vi "zmq_data_server.vi"() -> ()   [LabVIEW 2013]
doc: "Sends a specified waveform through a TCP port. The VI first listens for a connection and, once established, sends the number of bytes to be sent followed by the data. After the data is sent, the VI waits for an 'all received' signal from the client and then breaks the connection.\n\n<B>Note:</B> Requires the Data Client.vi located in the same library as this VI."
uses:
  <vilib>/addons/zeromq/socket_type.ctl
panel:
  in  "amplitude period (ms)":u32
  out "Waveform Graph":dbl[](graph)
  out "*(type *) &x":string
  in  "stop":bool
  in  "Noise Level":dbl(slide)=0.36734693877551017 scale=0.0..1.0 scale format="%0.1f"
  in  "# of Points":i32=200
  in  "Function":u16(ring)=1 items=["random", "sine wave", "cosine wave"]
  in  "Port":u16=6340 min=1025 step=1
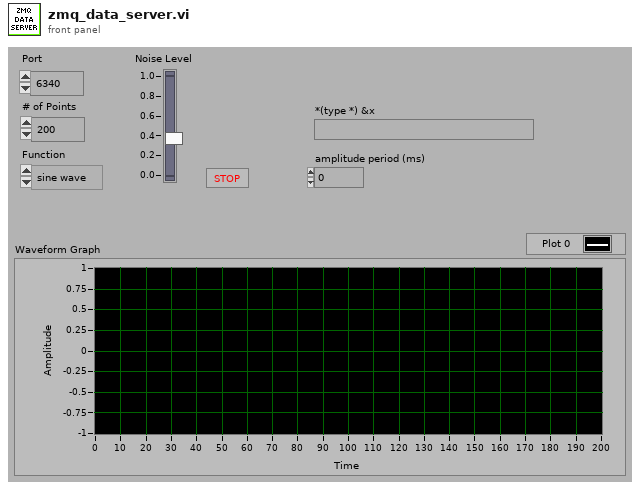
[diagram p1: front panel]
types:
  T1 = typedef "zeromq.lvlib/socket_type.ctl" = enum8{"ZMQ_PAIR", "ZMQ_PUB", "ZMQ_SUB", "ZMQ_REQ", "ZMQ_REP", "ZMQ_DEALER", "ZMQ_ROUTER", "ZMQ_PULL", "ZMQ_PUSH", "ZMQ_XPUB", "ZMQ_XSUB"}
  T2 = typedef "pointer.ctl" = u64
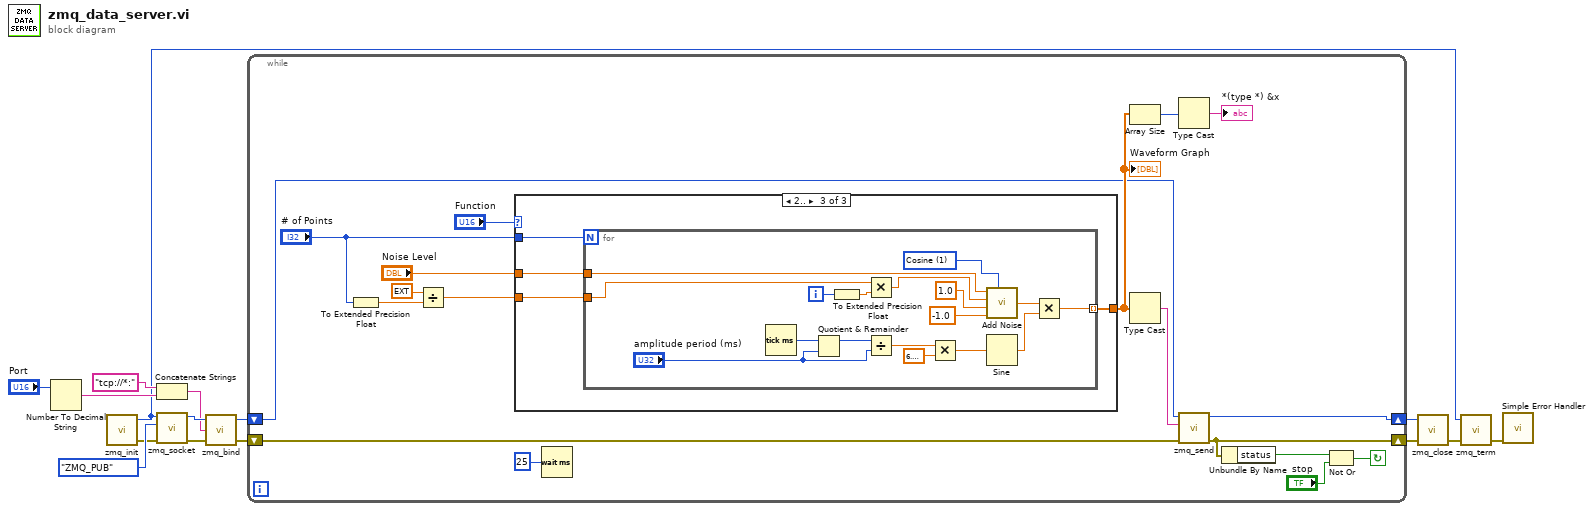
[diagram p0: block diagram]
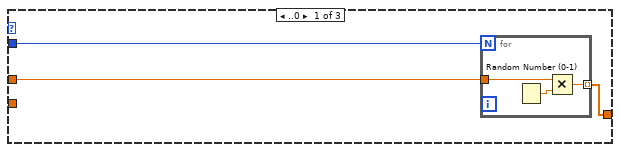
[diagram p2: hidden frame]
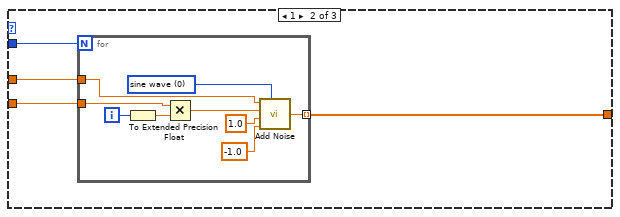
[diagram p3: hidden frame]
diagram:
  n1 = Number To Decimal String(number="Port") -> (decimal integer string=w8:string)  [unwired: 1 in]
  n2 = call <vilib>:"zmq_init.vi"() -> ("error out"=w14:errorcluster, "context"=w1:T2)  [unwired: 4 in]
  n3 = Concatenate Strings("tcp://*:" ("port"), w8) -> (w10:string)
  n4 = call <vilib>:"zmq_socket.vi"("error in"=w14, "socket type"=socket_type."ZMQ_PUB", "ctx in"=w1) -> ("error out"=w13:errorcluster, "socket"=w12:T2)  [unwired: 3 in]
  n5 = call <vilib>:"zmq_bind.vi"("error in"=w13, "endpoint"=w10, "socket in"=w12) -> ("error out"=w4:errorcluster, "socket out"=w3:T2)  [unwired: 1 in]
  n6 = while {
    shift-right: [w18] -> w2
    shift-left: w3 -> [w16]
    shift-right: [w20] -> w5
    shift-left: w4 -> [w17]
    stop <- w33 continue-if-true
    n7 = To Extended Precision Float(1:"# of Points") -> (0:w31:ext)
    n8 = Divide(x=ext 6.283185307179586477, y=w31) -> (x/y=w28:ext)
    n9 = case shown="2.." "Function" {
      tunnel: "# of Points" -> [w36 w43 w56]
      tunnel: [w35 w40 w53] -> w24
      tunnel: w28 -> [_ w42 w54]
      tunnel: "Noise Level" -> [w34 w41 w55]
      frame ..0 {
        n10 = for {
          N: w36 -> [_]
          tunnel: [w37] -> w35 mode=indexing
          tunnel: w34 -> [w39]
          n11 = Random Number (0-1)() -> (number: 0 to 1=w38:dbl)
          n12 = Multiply(x=w39, y=w38) -> (x*y=w37:dbl)
        }
      }
      frame 1 {
        n13 = for {
          N: w43 -> [_]
          tunnel: w42 -> [w51]
          tunnel: w41 -> [w50]
          tunnel: [w49] -> w40 mode=indexing
          i -> [w52]
          w44 = u16 0 items=["sine wave", "cosine wave"] ("Function")
          n14 = To Extended Precision Float(1:w52) -> (0:w48:ext)
          n15 = Multiply(x=w51, y=w48) -> (x*y=w45:ext)
          n16 = call "Add Noise.vi"("noise"=w50, "input"=w45, "max"=1.0, "min"=-1.0, "Function"=w44) -> ("output"=w49:dbl)
        }
      }
      frame 2.. {
        n17 = for {
          N: w56 -> [_]
          tunnel: w55 -> [w69]
          tunnel: w54 -> [w68]
          tunnel: [w61] -> w53 mode=indexing
          i -> [w73]
          w66 = u16 1 items=["Sine", "Cosine"] ("Function")
          n18 = Tick Count (ms)() -> (millisecond timer value=w65:u32)
          n19 = Quotient & Remainder(x=w65, y="amplitude period (ms)") -> (x-y*floor(x/y)=w64:u32)  [unwired: 1 out]
          n20 = To Extended Precision Float(1:w73) -> (0:w72:ext)
          n21 = Multiply(x=w68, y=w72) -> (x*y=w67:ext)
          n22 = Divide(x=w64, y="amplitude period (ms)") -> (x/y=w60:dbl)
          n23 = Multiply(x=w60, y=6.283185307179586) -> (x*y=w58:dbl)
          n24 = call "Add Noise.vi"("noise"=w69, "input"=w67, "max"=1.0, "min"=-1.0, "Function"=w66) -> ("output"=w62:dbl)
          n25 = Sine(x=w58) -> (sin(x)=w57:dbl)
          n26 = Multiply(x=w62, y=w57) -> (x*y=w61:dbl)
        }
      }
    }
    "Waveform Graph" <- w24
    n27 = Wait (ms)(milliseconds to wait=u32 25) -> ()  [unwired: 1 out]
    n28 = Array Size(array=w24) -> (size(s)=w23:i32)
    n29 = Type Cast(x=w24) -> (*(type *) &x=w22:string)  [unwired: 1 in]
    n30 = Type Cast(x=w23) -> (*(type *) &x=→"*(type *) &x":string)  [unwired: 1 in]
    n31 = call <vilib>:"zmq_send.vi"("error in"=w17, "data"=w22, "socket in"=w16) -> ("error out"=w20:errorcluster, "socket out"=w18:T2)  [unwired: 4 in]
    n32 = Unbundle By Name(w20) -> ("status"=w32:bool)
    n33 = Not Or(1:"stop", 2:w32) -> (0:w33:bool)
  }
  n34 = call <vilib>:"zmq_close.vi"("error in"=w5, "socket in"=w2) -> ("error out"=w7:errorcluster)  [unwired: 3 in]
  n35 = call <vilib>:"zmq_term.vi"("error in"=w7, "context"=w1) -> ("error out"=w6:errorcluster)  [unwired: 3 in]
  n36 = call <vilib>:"Simple Error Handler.vi"("error in (no error)"=w6) -> ()  [unwired: 4 in, 5 out]
